vi "SelectDailyDataAll.vi"(8 "Shift":string="中", 10 "End_date":string="2014/11/13", 11 "Begin_date":string="2014/11/12") -> (2 "output array":string[][](array[string]))   [LabVIEW 2012]
uses:
  <vilib>/addons/database/Auxilliary.llb/DB Tools Cursor Type.ctl
  <vilib>/addons/database/Connection.llb/DB Tools Open Connec (Path).vi
  <vilib>/addons/database/Connection.llb/Conn Execute.vi
  <vilib>/addons/database/Recordset.llb/Rec Fetch Recordset Data (R).vi
  <vilib>/addons/database/Recordset.llb/Rec Destroy - Connection.vi
  <vilib>/addons/database/_DB Variant To Data/Database Variant To Data.xnode
  <vilib>/addons/database/NI_Database_API.lvlib
panel:
  out "concatenated string":string
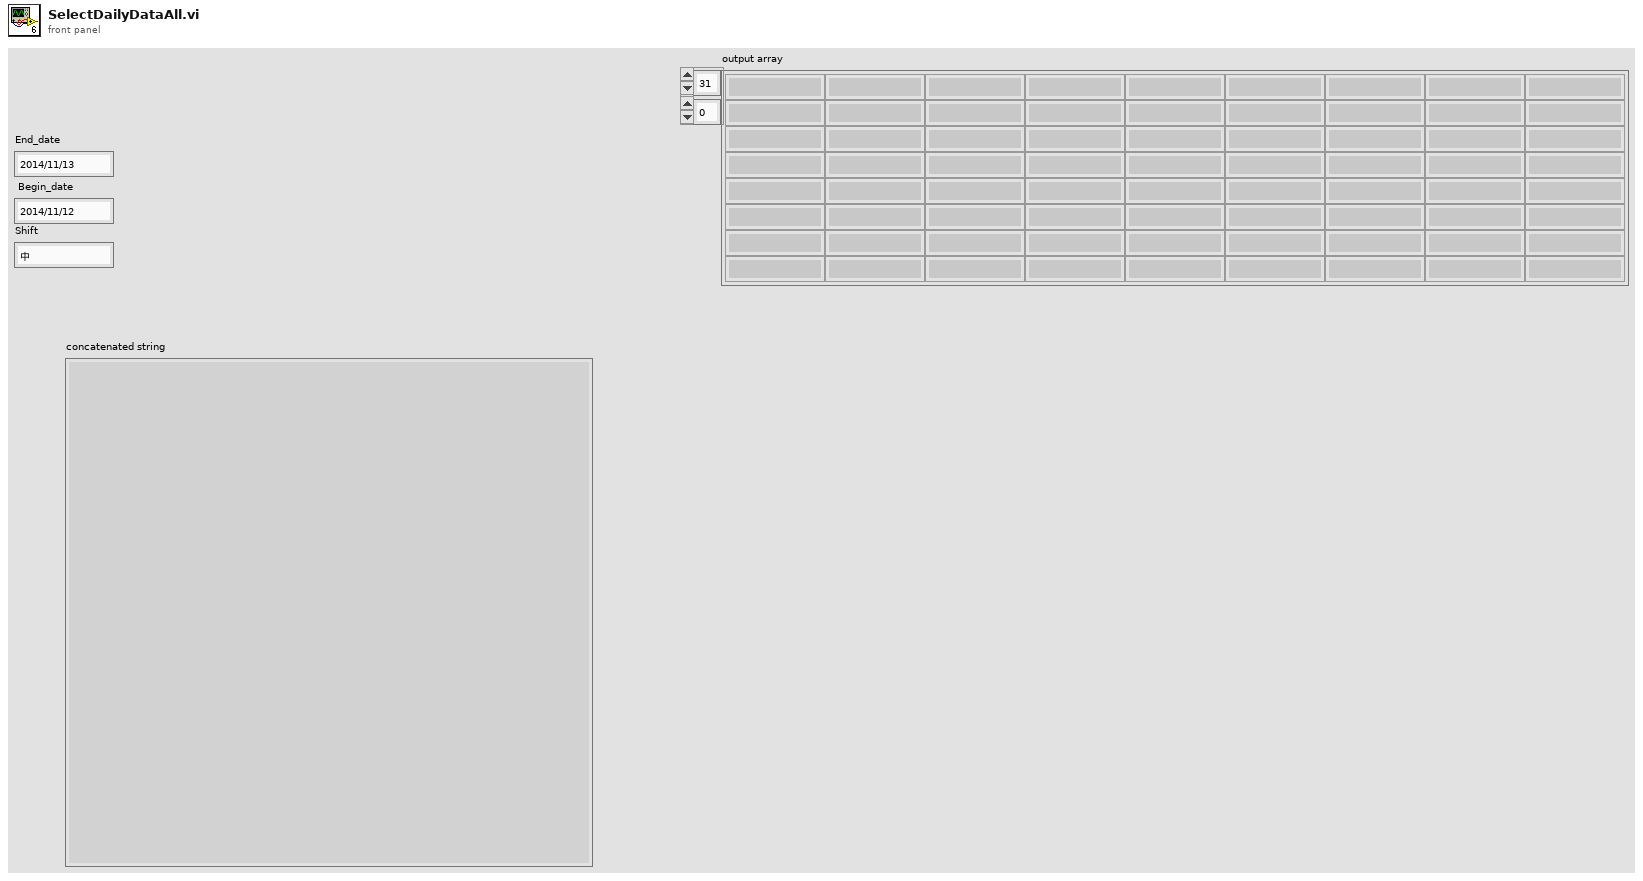
[diagram p1: front panel]
types:
  T1 = typedef "NI_Database_API.lvlib/DB Tools Cursor Type.ctl" = enum16{"forward-only", "keyset", "dynamic", "static"}
  T2 = typedef "NI_Database_API.lvlib/Conn ObjectReference.ctl" = refnum<k1>
  T3 = typedef "NI_Database_API.lvlib/Rec ObjectReference.ctl" = refnum<k1>
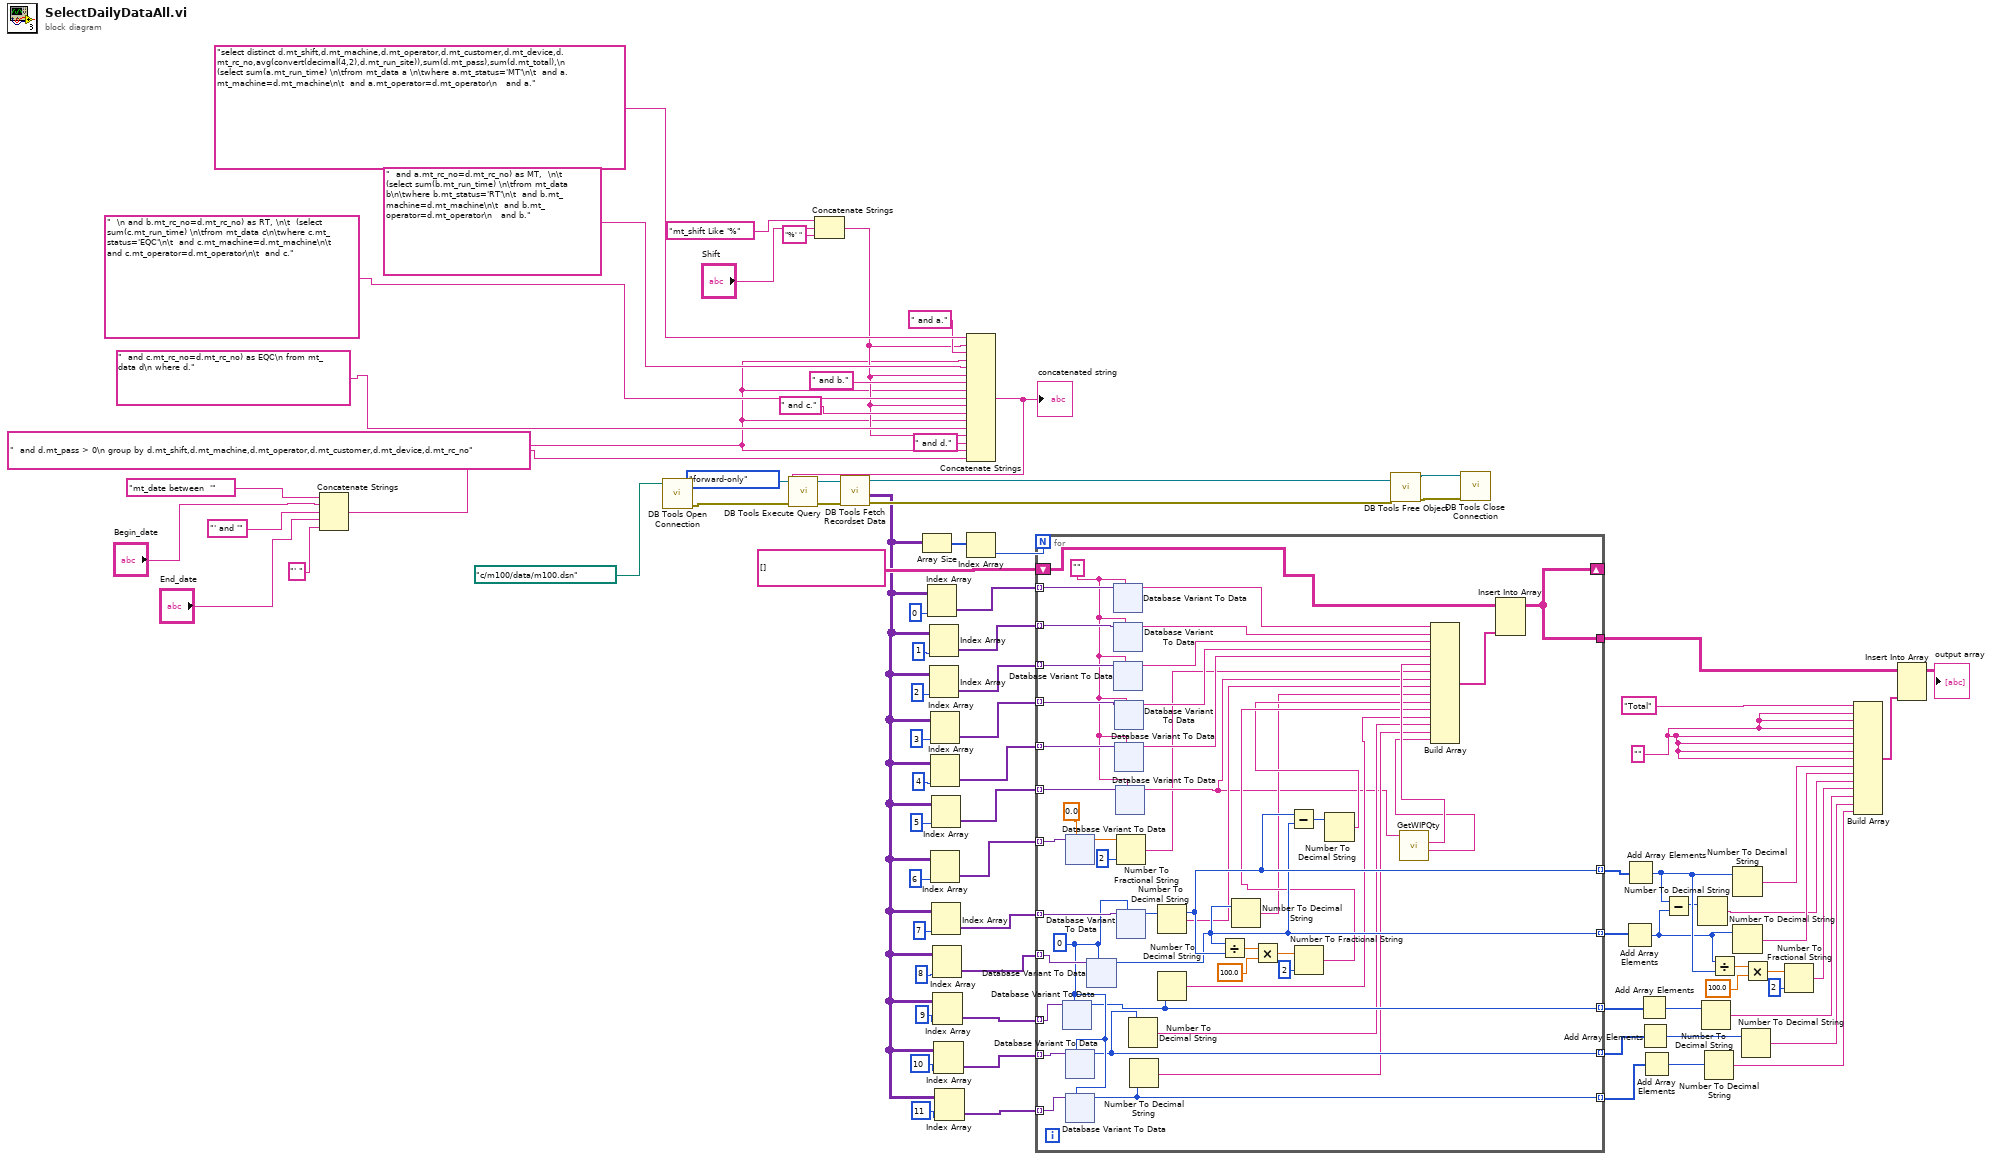
[diagram p0: block diagram]
diagram:
  w1 = "" ("element")
  n1 = Concatenate Strings("mt_date between  '", "Begin_date", "' and '" ("string"), "End_date", "' " ("string")) -> (w9:string)
  n2 = call-poly <vilib>:"DB Tools Open Connection.vi"("connection information"=path "c:/m100/data/m100.dsn") -> ("error out"=w53:errorcluster, "connection reference"=w54:T2)  [unwired: 7 in]
  n3 = Concatenate Strings("mt_shift Like '%" ("string"), "Shift", "%' " ("string")) -> (w11:string)
  n4 = Concatenate Strings("select distinct d.mt_shift,d.mt_machine,d.mt_operator,d.mt_customer,d.mt_device,d.mt_rc_no,avg(convert(decimal(4,2),d.mt_run_site)),sum(d.mt_pass),sum(d.mt_total),\n (select sum(a.mt_run_time) \n\tfrom mt_data a \n\twhere a.mt_status='MT'\n\t  and a.mt_machine=d.mt_machine\n\t  and a.mt_operator=d.mt_operator\n   and a." ("string"), w11, " and a." ("string"), w9, "  and a.mt_rc_no=d.mt_rc_no) as MT,  \n\t  (select sum(b.mt_run_time) \n\tfrom mt_data b\n\twhere b.mt_status='RT'\n\t  and b.mt_machine=d.mt_machine\n\t  and b.mt_operator=d.mt_operator\n   and b." ("string"), w11, " and b." ("string"), w9, "  \n and b.mt_rc_no=d.mt_rc_no) as RT, \n\t  (select sum(c.mt_run_time) \n\tfrom mt_data c\n\twhere c.mt_status='EQC'\n\t  and c.mt_machine=d.mt_machine\n\t  and c.mt_operator=d.mt_operator\n\t  and c." ("string"), w11, " and c." ("string"), w9, "  and c.mt_rc_no=d.mt_rc_no) as EQC\n from mt_data d\n where d." ("string"), w11, " and d." ("string"), w9, "  and d.mt_pass > 0\n group by d.mt_shift,d.mt_machine,d.mt_operator,d.mt_customer,d.mt_device,d.mt_rc_no" ("string")) -> (w50:string)
  "concatenated string" <- w50
  n5 = call-poly <vilib>:"DB Tools Execute Query.vi"("error in (no error)"=w53, "cursor type"=DB_Tools_Cursor_Type."forward-only", "SQL query"=w50, "connection reference"=w54) -> ("error out"=w56:errorcluster, "recordset reference"=w55:T3)  [unwired: 4 in]
  n6 = call-poly <vilib>:"DB Tools Fetch Recordset Data.vi"("error in (no error)"=w56, "recordset reference"=w55) -> ("error out"=w52:errorcluster, "recordset data"=w5:variant[][], "recordset reference out"=w51:T3)  [unwired: 3 in]
  n7 = Array Size(array=w5) -> (size(s)=w85:i32[])
  n8 = Index Array(array=w5, index (col)=0) -> (element=w74:variant[])  [unwired: 1 in]
  n9 = Index Array(array=w5, index (col)=1) -> (element=w81:variant[])  [unwired: 1 in]
  n10 = Index Array(array=w5, index (col)=2) -> (element=w73:variant[])  [unwired: 1 in]
  n11 = Index Array(array=w5, index (col)=3) -> (element=w72:variant[])  [unwired: 1 in]
  n12 = Index Array(array=w5, index (col)=4) -> (element=w71:variant[])  [unwired: 1 in]
  n13 = Index Array(array=w5, index (col)=6 ("disabled index (col)")) -> (element=w3:variant[])  [unwired: 1 in]
  n14 = Index Array(array=w5, index (col)=5) -> (element=w67:variant[])  [unwired: 1 in]
  n15 = Index Array(array=w5, index (col)=7) -> (element=w70:variant[])  [unwired: 1 in]
  n16 = Index Array(array=w5, index (col)=8) -> (element=w69:variant[])  [unwired: 1 in]
  n17 = Index Array(array=w5, index (col)=9) -> (element=w44:variant[])  [unwired: 1 in]
  n18 = Index Array(array=w5, index (col)=10) -> (element=w43:variant[])  [unwired: 1 in]
  n19 = Index Array(array=w5, index (col)=11) -> (element=w42:variant[])  [unwired: 1 in]
  n20 = Index Array(array=w85) -> (element=w84:i32)  [unwired: 1 in]
  n21 = for {
    N: w84 -> [_]
    tunnel: w81 -> [w129] mode=indexing
    tunnel: w69 -> [w131] mode=indexing
    shift-right: [w112] -> _
    shift-left: string[][] [] -> [w118]
    tunnel: w74 -> [w130] mode=indexing
    tunnel: w73 -> [w128] mode=indexing
    tunnel: w72 -> [w127] mode=indexing
    tunnel: w71 -> [w126] mode=indexing
    tunnel: w70 -> [w125] mode=indexing
    tunnel: w67 -> [w122] mode=indexing
    tunnel: [w104] -> w31 mode=indexing
    tunnel: [w103] -> w65 mode=indexing
    tunnel: [w112] -> w48
    tunnel: w44 -> [w111] mode=indexing
    tunnel: w43 -> [w110] mode=indexing
    tunnel: w42 -> [w109] mode=indexing
    tunnel: [w107] -> w39 mode=indexing
    tunnel: [w106] -> w40 mode=indexing
    tunnel: [w105] -> w41 mode=indexing
    tunnel: w3 -> [w100] mode=indexing
    w108 = 0
    w90 = ""
    n22 = xnode "Database Variant To Data"("database variant"=w111, "type"=w108) -> ("data"=w105:i32)  [unwired: 1 in, 1 out]
    n23 = xnode "Database Variant To Data"("database variant"=w100, "type"=0.0) -> ("data"=w88:dbl)  [unwired: 1 in, 1 out]
    n24 = xnode "Database Variant To Data"("database variant"=w110, "type"=w108) -> ("data"=w106:i32)  [unwired: 1 in, 1 out]
    n25 = xnode "Database Variant To Data"("database variant"=w109, "type"=w108) -> ("data"=w107:i32)  [unwired: 1 in, 1 out]
    n26 = xnode "Database Variant To Data"("database variant"=w131, "type"=w108) -> ("data"=w103:i32)  [unwired: 1 in, 1 out]
    n27 = xnode "Database Variant To Data"("database variant"=w130, "type"=w90) -> ("data"=w117:string)  [unwired: 1 in, 1 out]
    n28 = xnode "Database Variant To Data"("database variant"=w129, "type"=w90) -> ("data"=w116:string)  [unwired: 1 in, 1 out]
    n29 = xnode "Database Variant To Data"("database variant"=w128, "type"=w90) -> ("data"=w113:string)  [unwired: 1 in, 1 out]
    n30 = xnode "Database Variant To Data"("database variant"=w127, "type"=w90) -> ("data"=w115:string)  [unwired: 1 in, 1 out]
    n31 = xnode "Database Variant To Data"("database variant"=w126, "type"=w90) -> ("data"=w114:string)  [unwired: 1 in, 1 out]
    n32 = xnode "Database Variant To Data"("database variant"=w122, "type"=w90) -> ("data"=w91:string)  [unwired: 1 in, 1 out]
    n33 = Number To Fractional String(number=w88, precision (6)=i16 2) -> (F-format string=w87:string)  [unwired: 2 in]
    n34 = xnode "Database Variant To Data"("database variant"=w125, "type"=w108) -> ("data"=w104:i32)  [unwired: 1 in, 1 out]
    n35 = Number To Decimal String(number=w106) -> (decimal integer string=w97:string)  [unwired: 1 in]
    n36 = Number To Decimal String(number=w107) -> (decimal integer string=w98:string)  [unwired: 1 in]
    n37 = Number To Decimal String(number=w104) -> (decimal integer string=w92:string)  [unwired: 1 in]
    n38 = Number To Decimal String(number=w105) -> (decimal integer string=w96:string)  [unwired: 1 in]
    n39 = Divide(x=w103, y=w104) -> (x/y=w123:dbl)
    n40 = Number To Decimal String(number=w103) -> (decimal integer string=w93:string)  [unwired: 1 in]
    n41 = Multiply(x=w123, y=100.0) -> (x*y=w121:dbl)
    n42 = Subtract(x=w104, y=w103) -> (x-y=w102:i32)
    n43 = Number To Fractional String(number=w121, precision (6)=i16 2) -> (F-format string=w95:string)  [unwired: 2 in]
    n44 = Number To Decimal String(number=w102) -> (decimal integer string=w94:string)  [unwired: 1 in]
    n45 = call "GetWIPQty.vi"("Lotno"=w91) -> ("lotno"=w99:string, "Package"=w101:string)  [unwired: 2 in, 7 out]
    n46 = Build Array(w117, w116, w113, w115, w114, w101, w87, w91, w92, w93, w94, w95, w96, w97, w98, w99) -> (w119:string[])
    n47 = Insert Into Array(array=w118, new element=w119) -> (w112:string[][])  [unwired: 2 in]
  }
  n48 = call-poly <vilib>:"DB Tools Free Object.vi"("error in (no error)"=w52, "recordset reference"=w51) -> ("error out"=w57:errorcluster, "connection reference"=w58:T2)  [unwired: 8 in]
  n49 = call <vilib>:"DB Tools Close Connection.vi"("error in (no error)"=w57, "connection reference"=w58) -> ()  [unwired: 5 in, 1 out]
  n50 = Add Array Elements(numeric array=w65) -> (sum=w29:i32)
  n51 = Add Array Elements(numeric array=w31) -> (sum=w30:i32)
  n52 = Add Array Elements(numeric array=w41) -> (sum=w38:i32)
  n53 = Add Array Elements(numeric array=w40) -> (sum=w37:i32)
  n54 = Add Array Elements(numeric array=w39) -> (sum=w36:i32)
  n55 = Subtract(x=w30, y=w29) -> (x-y=w28:i32)
  n56 = Number To Decimal String(number=w28) -> (decimal integer string=w27:string)  [unwired: 1 in]
  n57 = Number To Decimal String(number=w38) -> (decimal integer string=w33:string)  [unwired: 1 in]
  n58 = Number To Decimal String(number=w36) -> (decimal integer string=w35:string)  [unwired: 1 in]
  n59 = Divide(x=w29, y=w30) -> (x/y=w61:dbl)
  n60 = Number To Decimal String(number=w30) -> (decimal integer string=w26:string)  [unwired: 1 in]
  n61 = Number To Decimal String(number=w29) -> (decimal integer string=w64:string)  [unwired: 1 in]
  n62 = Number To Decimal String(number=w37) -> (decimal integer string=w34:string)  [unwired: 1 in]
  n63 = Multiply(x=w61, y=100.0) -> (x*y=w60:dbl)
  n64 = Number To Fractional String(number=w60, precision (6)=i16 2) -> (F-format string=w32:string)  [unwired: 2 in]
  n65 = Build Array("Total", w1, w1, w1, w1, w1, w1, w1, w26, w64, w27, w32, w33, w34, w35) -> (w63:string[])
  n66 = Insert Into Array(array=w48, new element=w63) -> (→"output array":string[][])  [unwired: 2 in]
